vi "Render.vi"(8 "error in":errorcluster, 11 "class data in":refnum<class "Game.lvclass">) -> (0 "error out":errorcluster, 2 "quit out":bool, 3 "class data out":refnum<class "Game.lvclass">)   [LabVIEW 2010, in "Labricks.lvlib" / "Game.lvclass"]
uses:
  Game.lvclass
  Brick_class/Brick.lvclass
  Game.lvclass/Game.ctl
  BoundingBox_class/BoundingBox.lvclass
  Paddle_class/Paddle.lvclass
  RenderBase/SceneRoot_class/SceneRoot.lvclass
  Text_class/properties/Text/SetText.vi
  Text_class/Text.lvclass
  RenderBase/Sprite_class/Sprite.lvclass
  Ball_class/Ball.lvclass
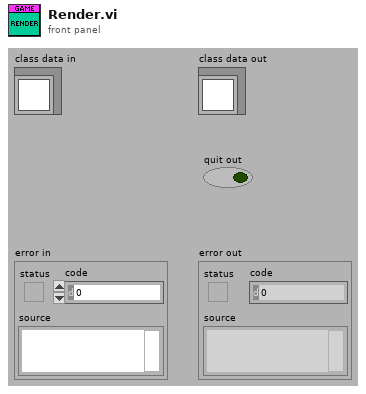
[diagram p1: front panel]
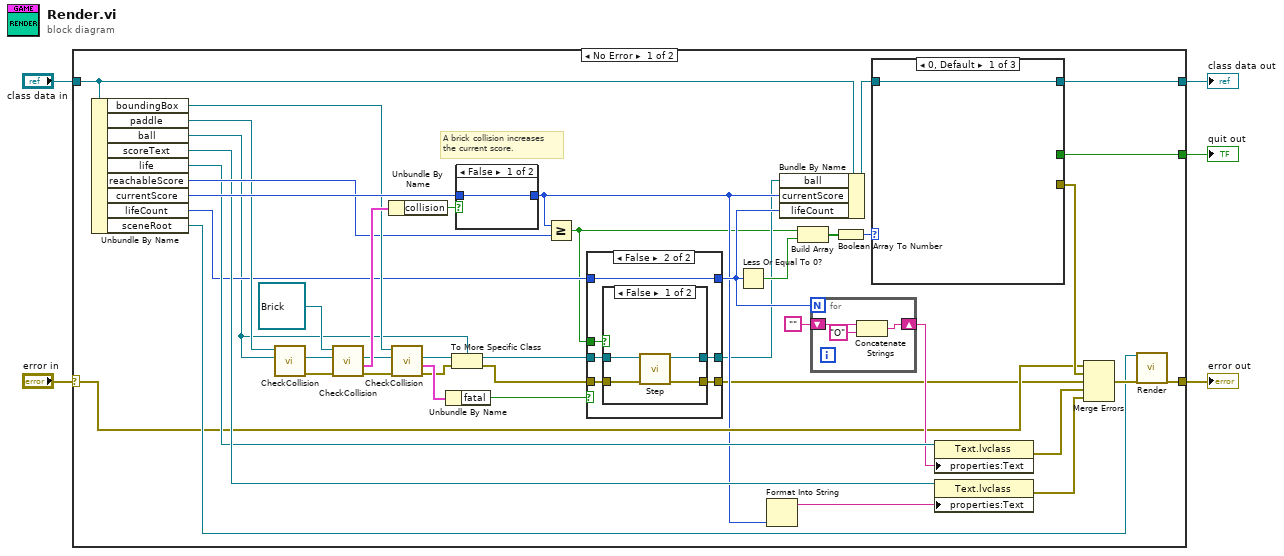
[diagram p0: block diagram]
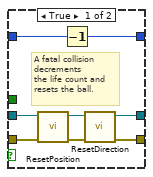
[diagram p2: hidden frame]
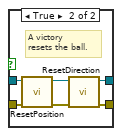
[diagram p3: hidden frame]
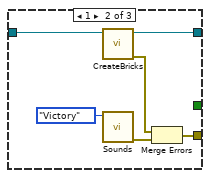
[diagram p4: hidden frame]
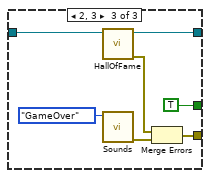
[diagram p5: hidden frame]
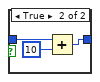
[diagram p6: hidden frame]
diagram:
  n1 = case shown="No Error" "error in" {
    selector: "error in" -> [w17 w95]
    tunnel: "class data in" -> [w21 w94]
    tunnel: [w19 w94] -> w2
    tunnel: [w40 w95] -> w3
    tunnel: [w18 _] -> w1
    frame No Error {
      # "A brick collision increases\nthe current score."
      n2 = Unbundle By Name(w21) -> ("boundingBox"=w43:refnum<class "BoundingBox.lvclass">, "paddle"=w37:refnum<class "Paddle.lvclass">, "ball"=w6:refnum<class "Ball.lvclass">, "scoreText"=w41:refnum<class "Text.lvclass">, "life"=w26:refnum<class "Text.lvclass">, "reachableScore"=w42:i32, "currentScore"=w44:i32, "lifeCount"=w15:i32, "sceneRoot"=w36:refnum<class "SceneRoot.lvclass">)
      n3 = call-dynamic "CheckCollision.vi"("sprite in"=w6, "class data in"=w37) -> ("error out"=w33:errorcluster, "sprite out"=w31:refnum<class "Sprite.lvclass">)  [unwired: 6 in, 2 out]
      n4 = call-dynamic "CheckCollision.vi"("error in"=w33, "sprite in"=w31, "class data in"=refnum<class "Brick.lvclass"> refnum ("brick in")) -> ("error out"=w32:errorcluster, "collisionInfo out"=w45:cluster{"collision":bool, "fatal":bool}, "sprite out"=w29:refnum<class "Sprite.lvclass">)  [unwired: 5 in, 1 out]
      n5 = Unbundle By Name(w45) -> ("collision"=w48:bool)
      n6 = call-dynamic "CheckCollision.vi"("error in"=w32, "sprite in"=w29, "class data in"=w43) -> ("error out"=w34:errorcluster, "collisionInfo out"=w47:cluster{"collision":bool, "fatal":bool}, "sprite out"=w35:refnum<class "Sprite.lvclass">)  [unwired: 5 in, 1 out]
      n7 = Unbundle By Name(w47) -> ("fatal"=w16:bool)
      n8 = To More Specific Class(target class=w6, reference=w35, error in=w34) -> (specific class reference=w11:refnum<class "Ball.lvclass">, error out=w10:errorcluster)
      n9 = case shown="False" w48 {
        tunnel: [w90 w91] -> w12
        tunnel: w44 -> [w90 w93]
        frame False {
        }
        frame True {
          n10 = Add(x=w93, y=10) -> (x+y=w91:i32)
        }
      }
      n11 = Greater Or Equal?(x=w12, y=w42) -> (x >= y?=w7:bool)
      n12 = case shown="False" w16 {
        tunnel: w15 -> [w56 w58]
        tunnel: [w55 w58] -> w14
        tunnel: w11 -> [w52 w62]
        tunnel: w10 -> [w51 w61]
        tunnel: [w50 w60] -> w9
        tunnel: [w49 w59] -> w8
        tunnel: w7 -> [_ w57]
        frame True {
          # "A fatal collision\ndecrements\nthe life count and\nresets the ball."
          n13 = call "ResetPosition.vi"("error in"=w51, "class data in"=w52) -> ("error out"=w54:errorcluster, "class data out"=w53:refnum<class "Ball.lvclass">)  [unwired: 8 in]
          n14 = Decrement(x=w56) -> (x-1=w55:i32)
          n15 = call "ResetDirection.vi"("error in"=w54, "class data in"=w53) -> ("error out"=w49:errorcluster, "class data out"=w50:refnum<class "Ball.lvclass">)  [unwired: 8 in]
        }
        frame False {
          n16 = case shown="False" w57 {
            tunnel: w62 -> [w64 w70]
            tunnel: w61 -> [w66 w69]
            tunnel: [w63 w68] -> w60
            tunnel: [w65 w67] -> w59
            frame False {
              n17 = call "Step.vi"("error in"=w66, "class data in"=w64) -> ("error out"=w65:errorcluster, "class data out"=w63:refnum<class "Ball.lvclass">)  [unwired: 8 in]
            }
            frame True {
              # "A victory\nresets the ball."
              n18 = call "ResetPosition.vi"("error in"=w69, "class data in"=w70) -> ("error out"=w72:errorcluster, "class data out"=w71:refnum<class "Ball.lvclass">)  [unwired: 8 in]
              n19 = call "ResetDirection.vi"("error in"=w72, "class data in"=w71) -> ("error out"=w67:errorcluster, "class data out"=w68:refnum<class "Ball.lvclass">)  [unwired: 8 in]
            }
          }
        }
      }
      n20 = Less Or Equal To 0?(x=w14) -> (x <= 0?=w13:bool)
      n21 = Format Into String(w12) -> (resulting string=w46:string)  [unwired: 3 in, 1 out]
      n22 = Bundle By Name(cluster=w21, "ball"=w9, "currentScore"=w12, "lifeCount"=w14) -> (w20:refnum<class "Game.lvclass">)
      n23 = Build Array(w7, w13) -> (w38:bool[])
      n24 = for {
        N: w14 -> [_]
        shift-right: [w88] -> w25
        shift-left: "" -> [w89]
        n25 = Concatenate Strings(w89, "O" ("string")) -> (w88:string)
      }
      n26 = Boolean Array To Number(Boolean array=w38) -> (number=w23:u32)
      n27 = case shown="0, Default" w23 {
        tunnel: w20 -> [w73 w79 w81]
        tunnel: [w73 w78 w80] -> w19
        tunnel: [_ w75 w84] -> w22
        tunnel: [_ _ TRUE] -> w18
        frame 0, Default {
        }
        frame 1 {
          n28 = call "CreateBricks.vi"("class data in"=w79) -> ("error out"=w77:errorcluster, "class data out"=w78:refnum<class "Game.lvclass">)  [unwired: 9 in]
          n29 = call "Sounds.vi"("choice in"=enum16{"Victory", "GameOver"}."Victory") -> ("error out"=w74:errorcluster)  [unwired: 10 in]
          n30 = Merge Errors(w77, w74) -> (w75:errorcluster)
        }
        frame 2, 3 {
          n31 = call "HallOfFame.vi"("class data in"=w81) -> ("error out"=w85:errorcluster, "class data out"=w80:refnum<class "Game.lvclass">)  [unwired: 9 in]
          n32 = call "Sounds.vi"("choice in"=enum16{"Victory", "GameOver"}."GameOver") -> ("error out"=w83:errorcluster)  [unwired: 10 in]
          n33 = Merge Errors(w85, w83) -> (w84:errorcluster)
        }
      }
      n34 = property class="Text.lvclass"(reference=w26, "properties:Text"=w25) -> (error out=w27:errorcluster)  [unwired: 1 in, 1 out]
      n35 = property class="Text.lvclass"(reference=w41, "properties:Text"=w46) -> (error out=w28:errorcluster)  [unwired: 1 in, 1 out]
      n36 = Merge Errors(w17, w22, w8, w27, w28) -> (w39:errorcluster)
      n37 = call-dynamic "Render.vi"("class data in"=w36, "error in (no error)"=w39) -> ("error out"=w40:errorcluster)  [unwired: 16 in, 1 out]
    }
    frame Error {
    }
  }
  "class data out" <- w2
  "error out" <- w3
  "quit out" <- w1
